vi "ControllingLED0.vi"() -> ()   [LabVIEW 2012]
panel:
  in  "LED0":bool
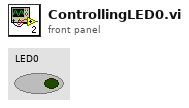
[diagram p1: front panel]
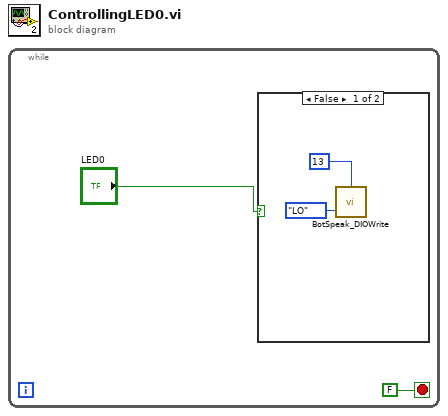
[diagram p0: block diagram]
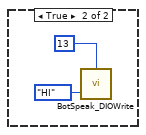
[diagram p2: hidden frame]
diagram:
  n1 = while {
    stop <- FALSE stop-if-true
    n2 = case shown="False" "LED0" {
      frame False {
        n3 = call <userlib>:"BotSpeak_DIOWrite.vi"("State"=enum32{"LO", "HI"}."LO", "DIO Line"=u32 13) -> ()  [unwired: 1 in, 2 out]
      }
      frame True {
        n4 = call <userlib>:"BotSpeak_DIOWrite.vi"("State"=enum32{"LO", "HI"}."HI", "DIO Line"=u32 13) -> ()  [unwired: 1 in, 2 out]
      }
    }
  }
